vi "PicoScope3000aSetRapidSegments.vi"(5 "RapidBlock":bool=TRUE, 7 "nSegments":T1 format="%.4p", 8 "error in (no error)":errorcluster, 11 "handle in":i16) -> (0 "error out":errorcluster, 3 "handle out":i16, 6 "nCaptures":u64)   [LabVIEW 2010]
doc: "Calls MemorySegments, and SetNoOfCaptures"
uses:
  ps3000a.dll
  shared/nSegments.ctl
panel:
  out "nMaxSamples":u64
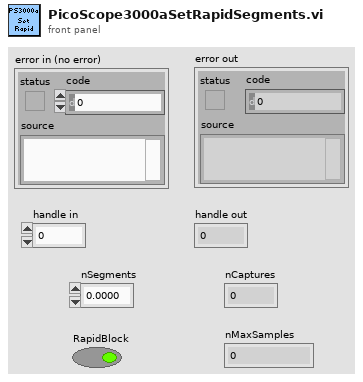
[diagram p1: front panel]
types:
  T1 = typedef "nSegments.ctl" = u64
  T2 = cluster{"status":bool, "code":u32, "source":string}
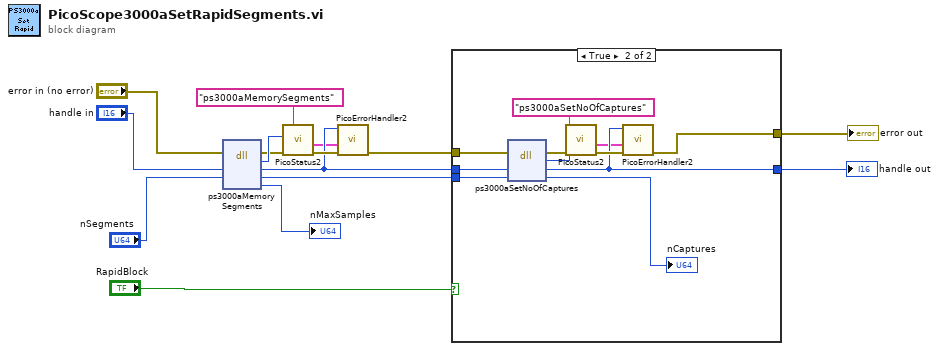
[diagram p0: block diagram]
diagram:
  n1 = dll-call lib="ps3000a.dll" fn="ps3000aMemorySegments" ("ps3000.dll:_ps3000_open_unit@0")(error in="error in (no error)", "handle"="handle in", "nSegments"="nSegments") -> (error out=w14:errorcluster, "PICO_STATUS"=w15:u32, "handle"=w10:i16, "nSegments"=w12:u32, "nMaxSamples"=→"nMaxSamples":i32)  [unwired: 3 in, 1 out]
  n2 = call "PicoStatus2.vi"("PICO source"="ps3000aMemorySegments" ("source"), "Error in"=w14, "PICO STATUS"=w15) -> ("error out"=w11:errorcluster, "PICO_STATUS out"=w1:T2)  [unwired: 5 in]
  n3 = call "PicoErrorHandler2.vi"("error in (no error)"=w11, "PICO_STATUS in"=w1, "handle In"=w10) -> ("error out"=w8:errorcluster)  [unwired: 8 in]
  n4 = case shown="True" "RapidBlock" {
    tunnel: w12 -> [_ w28]
    tunnel: w10 -> [w16 w25]
    tunnel: w8 -> [w17 w22]
    tunnel: [w17 w21] -> w5
    tunnel: [w16 w20] -> w4
    frame False {
    }
    frame True {
      n5 = dll-call lib="ps3000a.dll" fn="ps3000aSetNoOfCaptures" ("ps3000.dll:_ps3000_open_unit@0")(error in=w22, "handle"=w25, "nCaptures"=w28) -> (error out=w27:errorcluster, "PICO_STATUS"=w23:u32, "handle"=w20:i16, "nCaptures"=→"nCaptures":u32)  [unwired: 2 in, 1 out]
      n6 = call "PicoStatus2.vi"("PICO source"="ps3000aSetNoOfCaptures" ("source"), "Error in"=w27, "PICO STATUS"=w23) -> ("error out"=w24:errorcluster, "PICO_STATUS out"=w18:T2)  [unwired: 5 in]
      n7 = call "PicoErrorHandler2.vi"("error in (no error)"=w24, "PICO_STATUS in"=w18, "handle In"=w20) -> ("error out"=w21:errorcluster)  [unwired: 8 in]
    }
  }
  "error out" <- w5
  "handle out" <- w4
